vi "Stop Video.vi"(8 "error in (no error)":errorcluster, 11 "handle in":i64) -> (0 "error out":errorcluster, 2 "result":i32, 3 "handle out":i64)   [LabVIEW 2015]
uses:
  libkinect_wrapper.dll
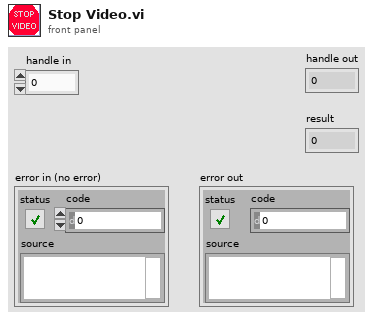
[diagram p1: front panel]
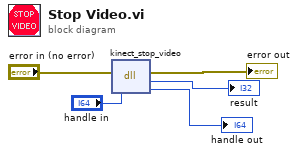
[diagram p0: block diagram]
diagram:
  n1 = dll-call lib="libkinect_wrapper.*" fn="kinect_stop_video"(error in="error in (no error)", "handle"="handle in") -> (error out=→"error out":errorcluster, "return type"=→"result":i32, "handle"=→"handle out":i64)  [unwired: 2 in, 1 out]
